vi "AgilentTest.vi"(11 "Adress":refnum<visa-resource-name>) -> (3 "Measurement":dbl)   [LabVIEW 2014]
uses:
  Agilent34401A/FGV.ctl
  Agilent34401A/Agilent34401AData.ctl
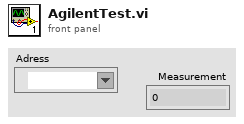
[diagram p1: front panel]
types:
  T1 = typedef "Agilent34401AData.ctl" = cluster{"Adress":refnum<visa-resource-name>}
  T2 = typedef "FGV.ctl" = enum16{"Write", "Read", "Init"}
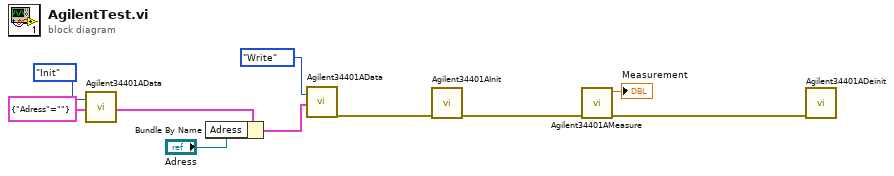
[diagram p0: block diagram]
diagram:
  n1 = call "Agilent34401AData.vi"("Enum"=FGV."Init", "Cluster"=T1 {"Adress"=""}) -> ("Cluster 2"=w4:T1)  [unwired: 16 in, 1 out]
  n2 = Bundle By Name(cluster=w4, "Adress"="Adress") -> (w3:T1)
  n3 = call "Agilent34401AData.vi"("Enum"=FGV."Write", "Cluster"=w3) -> ("error out"=w9:errorcluster)  [unwired: 16 in, 1 out]
  n4 = call "Agilent34401AInit.vi"("error in (no error)"=w9) -> ("error out"=w8:errorcluster)  [unwired: 10 in]
  n5 = call "Agilent34401AMeasure.vi"("error in (no error)"=w8) -> ("error out"=w7:errorcluster, "Measurement"=→"Measurement":dbl)  [unwired: 9 in]
  n6 = call "Agilent34401ADeinit.vi"("error in (no error)"=w7) -> ()  [unwired: 10 in, 1 out]
